vi "TDMS - File Viewer_Will.vi"(4 "error in (no error)":errorcluster, 7 "file path":path) -> (0 "error out":errorcluster, 3 "file path out":path)   [LabVIEW 2011]
doc: "Opens the .tdms file specified in the <B>file path</B> input and presents the file data in the TDMS File Viewer dialog box."
uses:
  <vilib>/Utility/tdmsutil.llb/fileViewerConfigData.ctl
  <vilib>/Utility/error.llb/DialogType.ctl
  <vilib>/Utility/tdmsutil.llb/TDMSFileViewerLocalizedText.vi
  Instance           1 26Saved   TDMS - File Viewer .vi
panel:
  in  "Help":bool
  in  "Status":string
  in  "Quit":bool
  in  "Settings...":bool
  in  "Properties / Values / Graph":T1(tab)
  in  "Properties":i32(listbox)
  in  "Raw data values":i32(listbox)
  out "Waveform Graph":waveform(dbl)[](graph)
  in  "File contents":string(tree)
  # "Displaying values 1..1000"
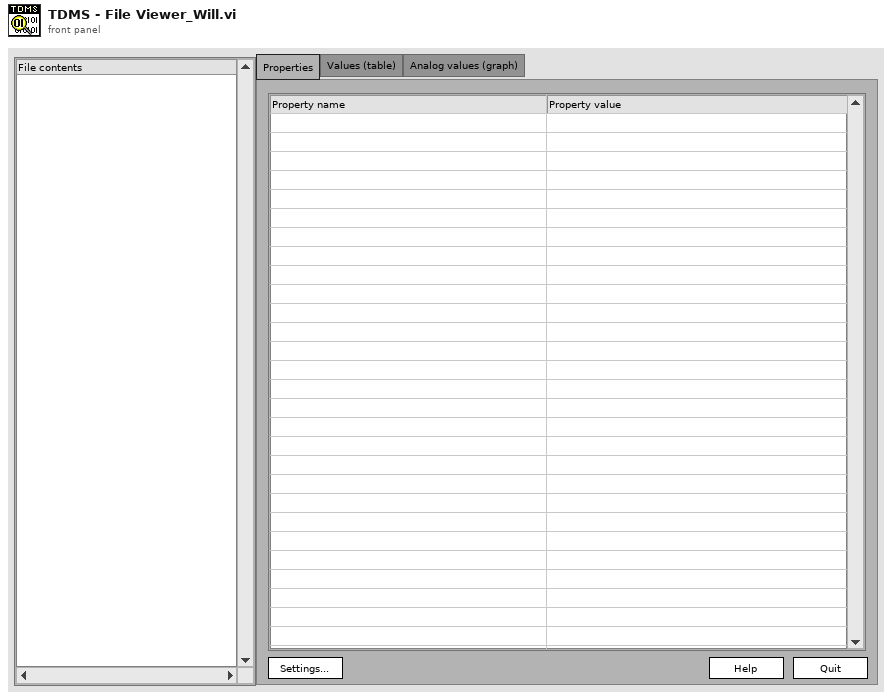
[diagram p1: front panel]
types:
  T1 = enum32{"Properties", "Values (table)", "Analog values (graph)"}
  T2 = enum16{"open", "open or create", "create or replace", "create", "open (read-only)"}
  T3 = cluster{"Tree":refnum<vi>, "Tab Control":refnum<vi>, "property list":refnum<vi>, "raw data list":refnum<vi>, "Waveform Graph":refnum<vi>, "Ok":refnum<vi>, "Ok 2":refnum<vi>, "Ok 3":refnum<vi>, "Ok 4":refnum<vi>}
  T4 = typedef "fileViewerConfigData.ctl" = cluster{"Show all (table)":bool, "Show all (graph)":bool, "limit (table)":u64, "limit (graph)":u64, "no show":bool, "start (table)":u64, "start (graph)":u64}
  T5 = typedef "DialogType.ctl" = u16
  T6 = typedef "LVRectTypeDef.ctl" = cluster{"left":i16, "top":i16, "right":i16, "bottom":i16}
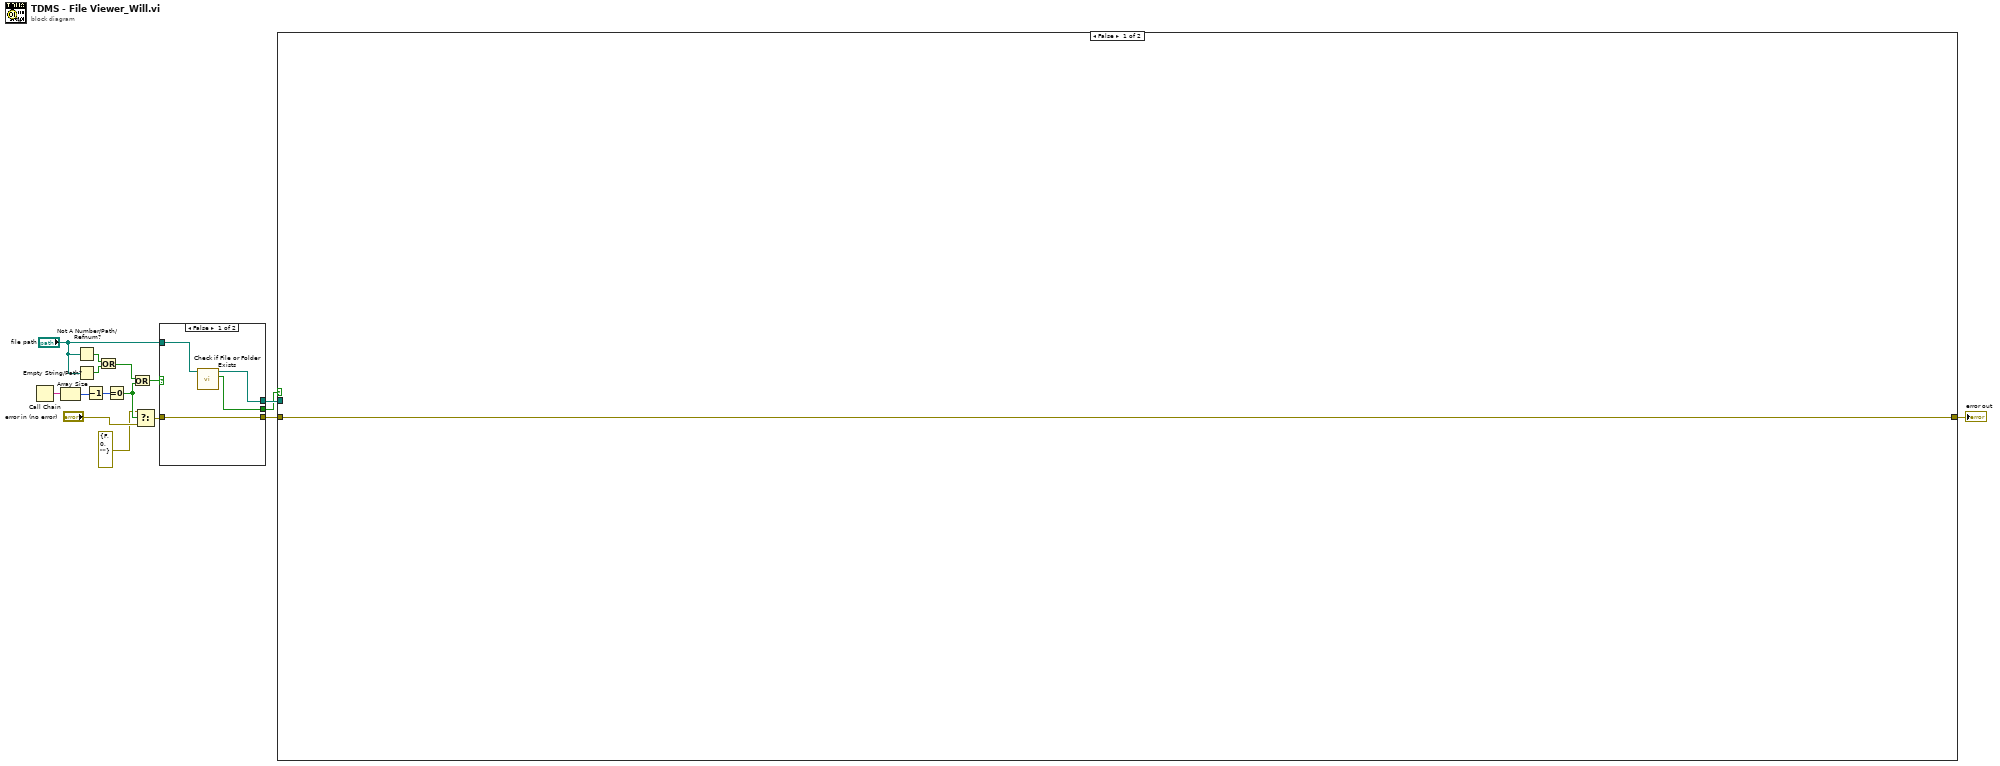
[diagram p0: block diagram]
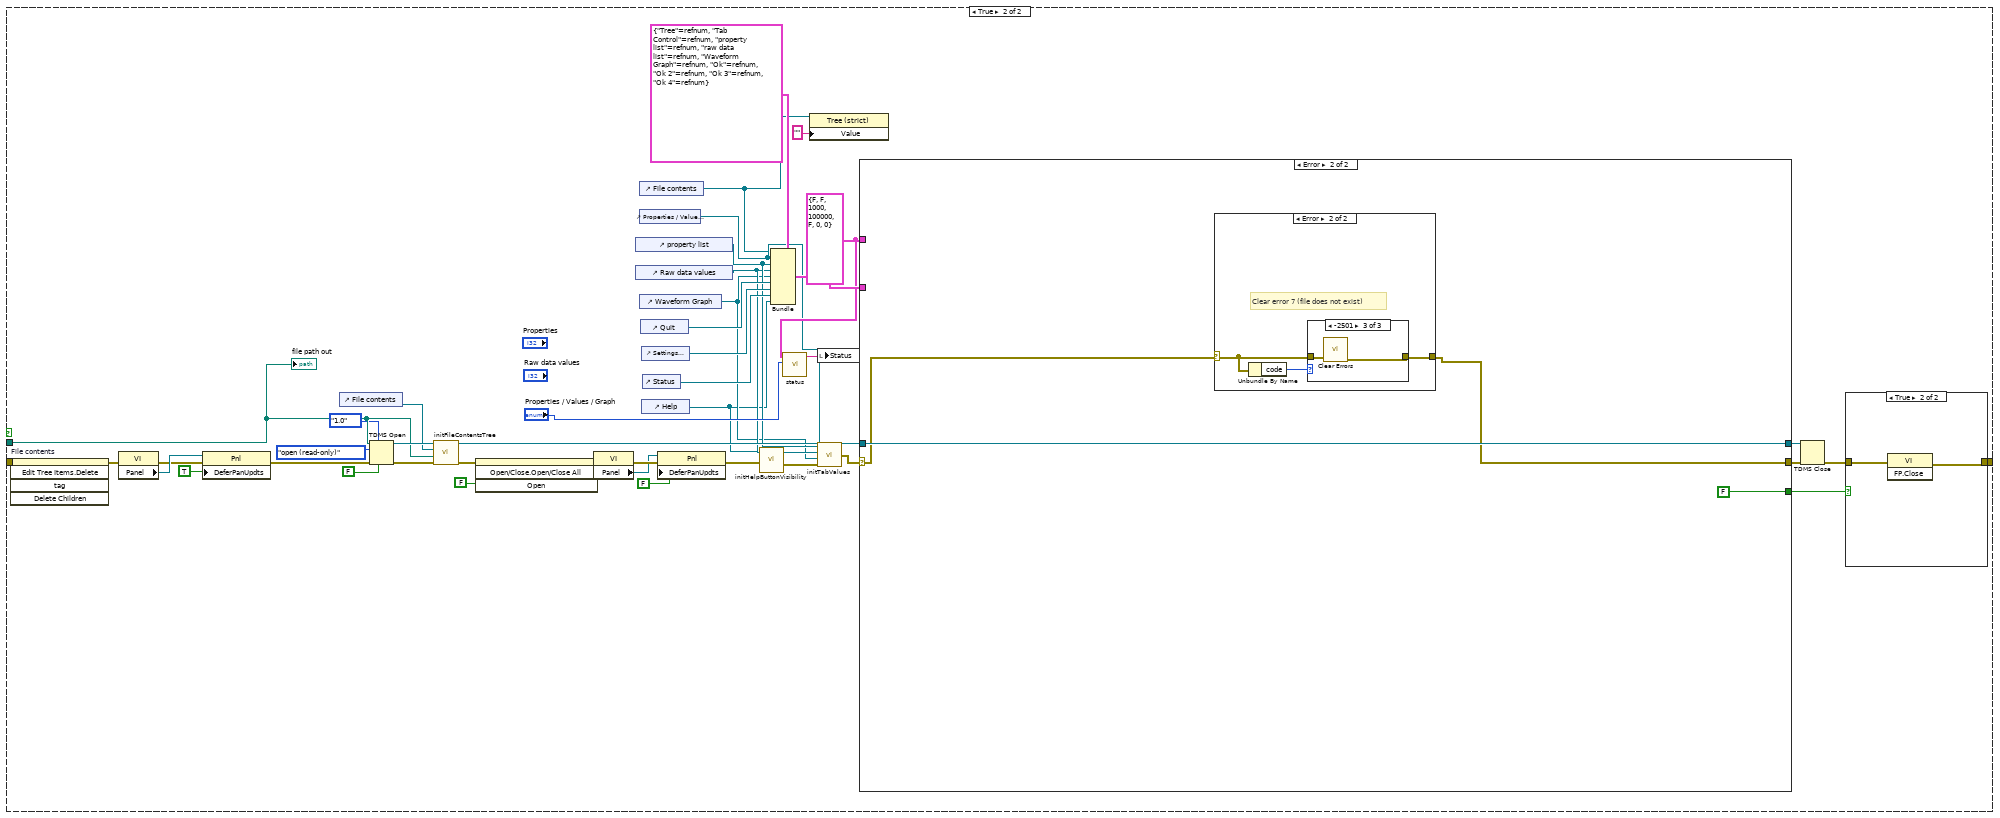
[diagram p2: hidden frame]
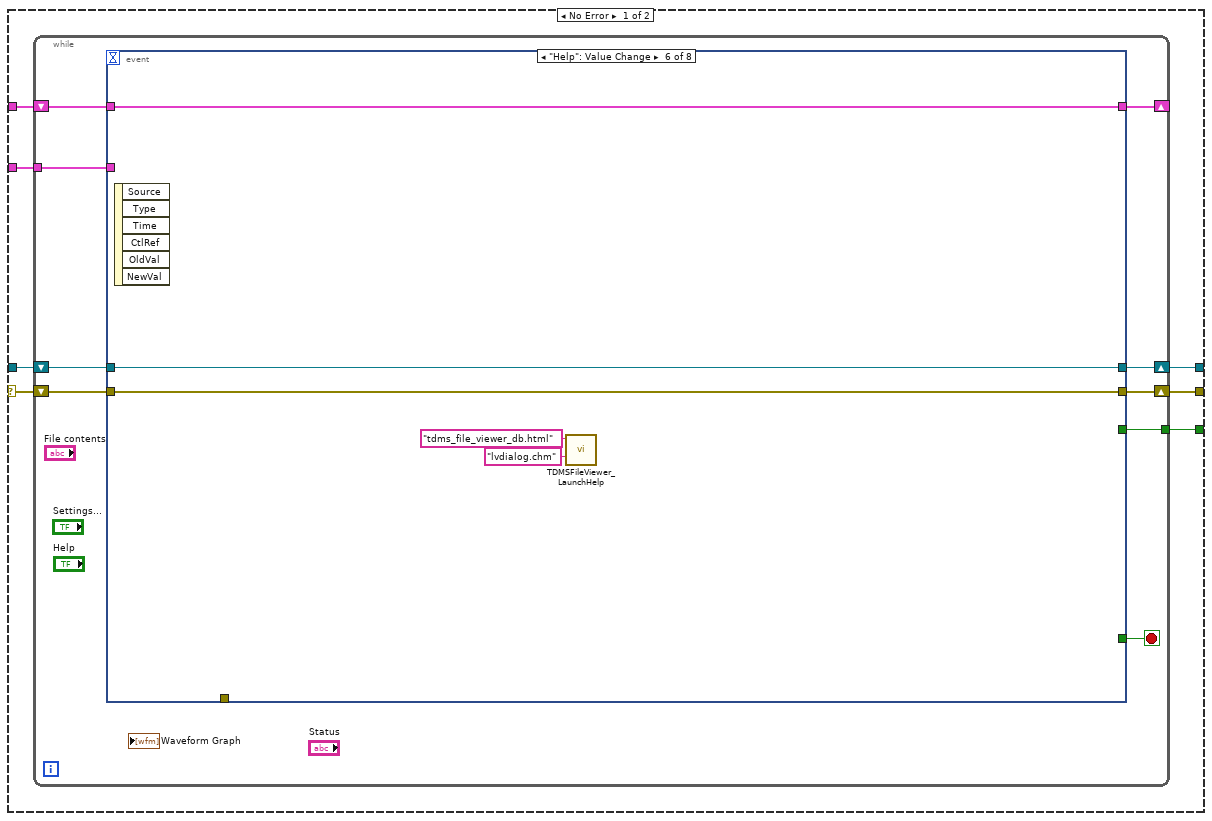
[diagram p4: hidden frame]
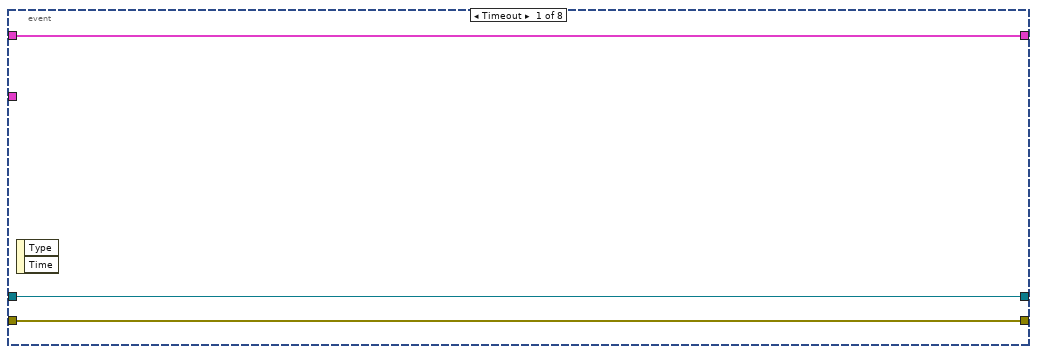
[diagram p5: hidden frame]
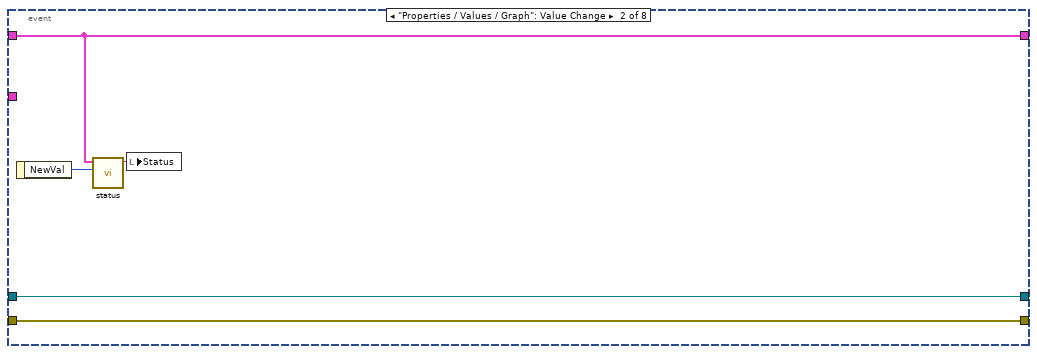
[diagram p6: hidden frame]
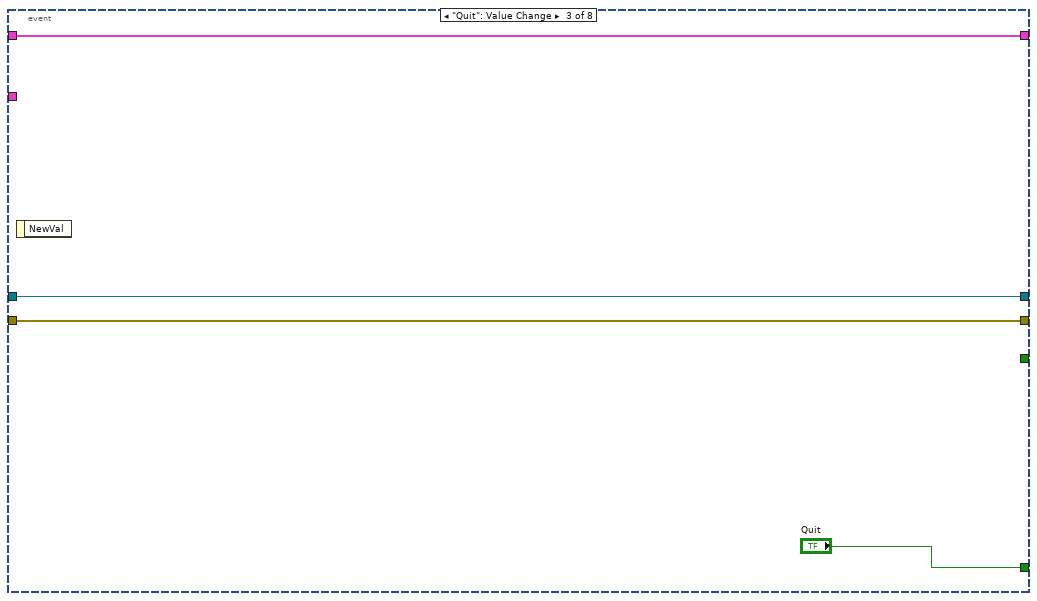
[diagram p7: hidden frame]
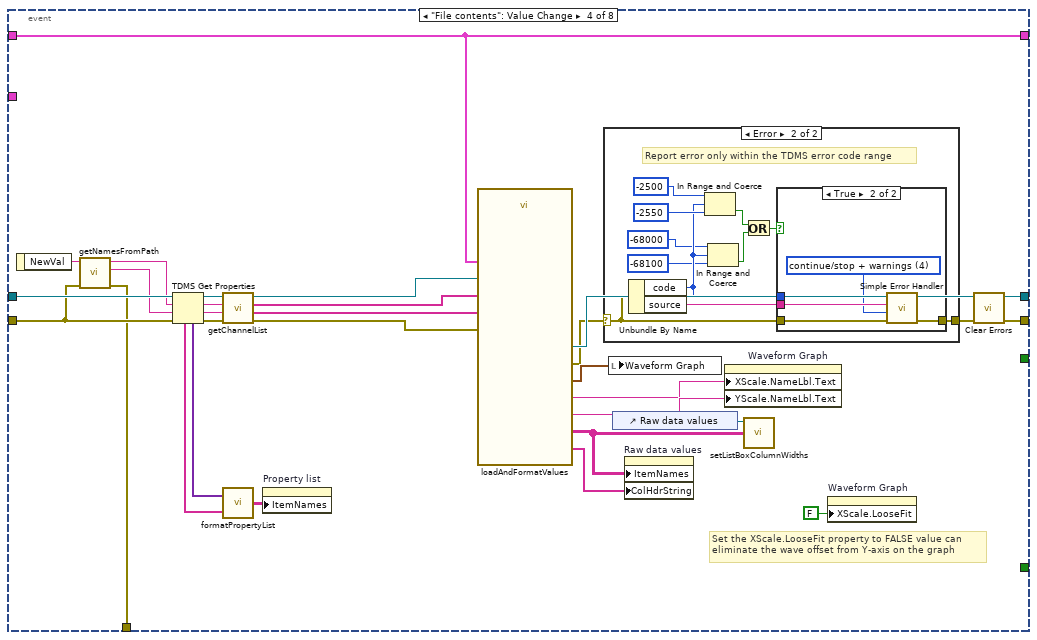
[diagram p8: hidden frame]
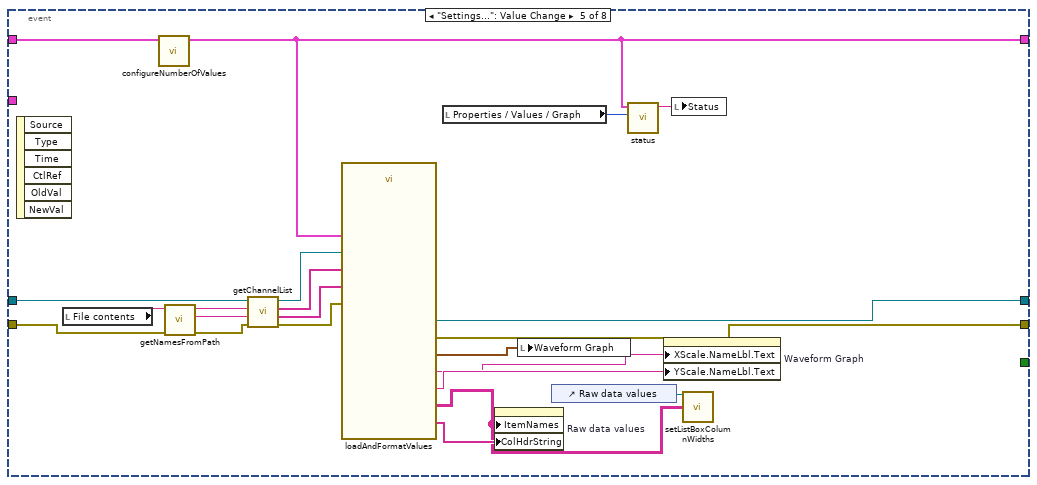
[diagram p11: hidden frame]
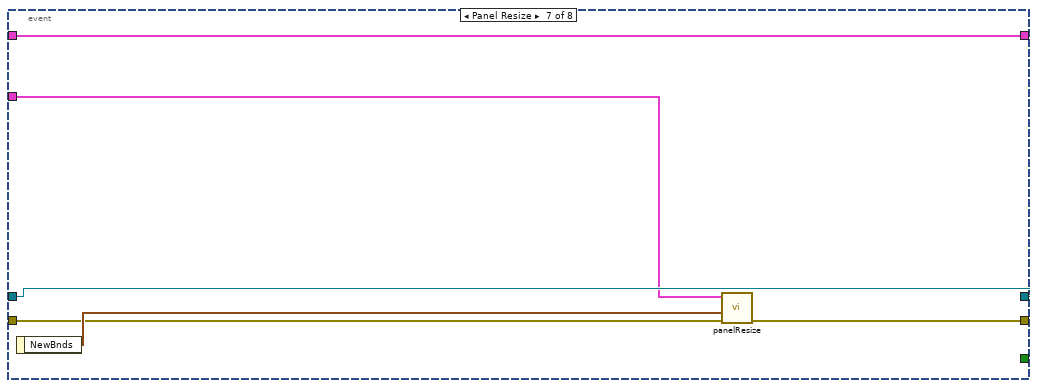
[diagram p12: hidden frame]
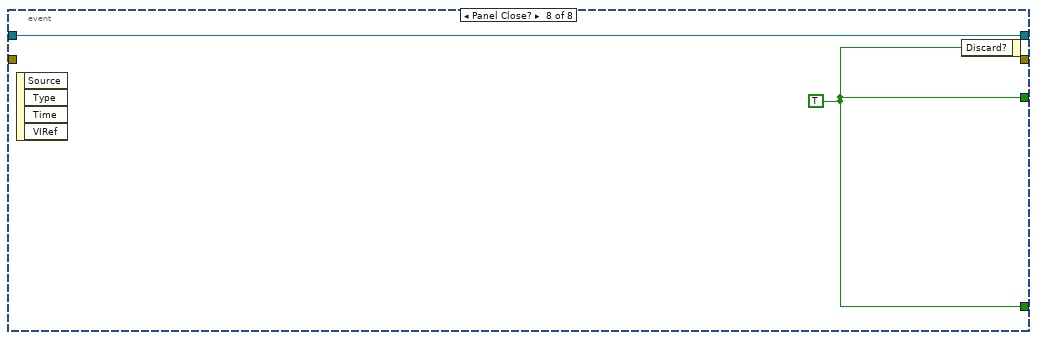
[diagram p13: hidden frame]
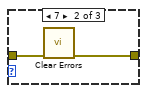
[diagram p16: hidden frame]
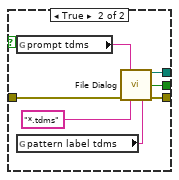
[diagram p17: hidden frame]
diagram:
  n1 = Call Chain() -> (call chain=w13:string[])
  n2 = Array Size(array=w13) -> (size(s)=w11:i32)
  n3 = Not A Number/Path/Refnum?(number/path/refnum="file path") -> (NaN/Path/Refnum?=w15:bool)
  n4 = Empty String/Path?(string/path="file path") -> (empty?=w14:bool)
  n5 = Decrement(x=w11) -> (x-1=w10:i32)
  n6 = Or(x=w15, y=w14) -> (x .or. y?=w12:bool)
  n7 = Equal To 0?(x=w10) -> (x = 0?=w6:bool)
  n8 = Or(x=w12, y=w6) -> (x .or. y?=w9:bool)
  n9 = Select(t=errorcluster {"status"=FALSE, "code"=0, "source"=""}, s=w6, f="error in (no error)") -> (s? t:f=w5:errorcluster)
  n10 = case shown="False" w9 {
    tunnel: [w18 w27] -> w8
    tunnel: "file path" -> [w19 _]
    tunnel: [w20 w25] -> w7
    tunnel: w5 -> [w20 w24]
    tunnel: [w17 w21] -> w1
    frame False {
      n11 = call <vilib>:"Check if File or Folder Exists.vi"("path"=w19) -> ("file or folder exists?"=w17:bool, "dup path"=w18:path)  [unwired: 8 in, 1 out]
    }
    frame True {
      n12 = global read "TDMSFileViewerLocalizedText.vi" "prompt tdms"() -> (w23:string)
      n13 = global read "TDMSFileViewerLocalizedText.vi" "pattern label tdms"() -> (w22:string)
      n14 = call "File Dialog"("prompt"=w23, "error in"=w24, "pattern (all files)"="*.tdms", "pattern label"=w22) -> ("selected path"=w27:path, "exists"=w21:bool, "error out"=w25:errorcluster)  [unwired: 3 in, 6 out]
    }
  }
  n15 = case shown="False" w1 {
    tunnel: w8 -> [_ w49]
    tunnel: w7 -> [w28 w48]
    tunnel: [w28 w41] -> w2
    frame False {
    }
    frame True {
      w45 = T4 {"Show all (table)"=FALSE, "Show all (graph)"=FALSE, "limit (table)"=1000, "limit (graph)"=100000, "no show"=FALSE, "start (table)"=0, "start (graph)"=0} ("TDMS File Viewer Configuration")
      n16 = invoke on="File contents" class="Tree (strict)" method="Edit Tree Items.Delete"(error in=w48) -> (error out=w62:errorcluster)  [unwired: 4 in, 4 out]
      n17 = property class="VI"(error in=w62) -> (error out=w63:errorcluster, "Panel"=w64:refnum<vi>)  [unwired: 1 in, 1 out]
      n18 = property class="Pnl"(reference=w64, error in=w63, "DeferPanUpdts"=TRUE ("Defer Panel Updates")) -> (error out=w66:errorcluster)  [unwired: 1 out]
      n19 = control-ref of="File contents"() -> (w50:refnum<vi>)
      n20 = TDMS Open(6:FALSE ("disable buffering (T)"), 7:enum16{"1.0", "2.0"}."1.0" ("file format version (2.0)"), 8:w66, 10:T2."open (read-only)" ("operation"), 11:w49) -> (0:w71:errorcluster, 3:w70:refnum<k34>)  [unwired: 1 in]
      n21 = call <vilib>:"initFileContentsTree.vi"("error in (no error)"=w71, "file path"=w49, "Tree Refnum"=w50, "tdms file"=w70) -> ("error out"=w58:errorcluster, "tdms file out"=w69:refnum<k34>)  [unwired: 2 out]
      n22 = invoke on="File contents" class="Tree (strict)" method="Open/Close.Open/Close All"(error in=w58, "Open"=FALSE ("Open?")) -> (error out=w57:errorcluster)  [unwired: 2 in, 3 out]
      n23 = property class="VI"(error in=w57) -> (error out=w60:errorcluster, "Panel"=w59:refnum<vi>)  [unwired: 1 in, 1 out]
      n24 = control-ref of="property list"() -> (w37:refnum<vi>)
      n25 = control-ref of="Raw data values"() -> (w36:refnum<vi>)
      n26 = control-ref of="Properties / Values / Graph"() -> (w34:refnum<vi>)
      n27 = control-ref of="Waveform Graph"() -> (w35:refnum<vi>)
      n28 = control-ref of="File contents"() -> (w33:refnum<vi>)
      n29 = control-ref of="Quit"() -> (w54:refnum<vi>)
      n30 = control-ref of="Settings..."() -> (w52:refnum<vi>)
      n31 = control-ref of="Help"() -> (w29:refnum<vi>)
      n32 = control-ref of="Status"() -> (w47:refnum<vi>)
      n33 = property class="Pnl"(reference=w59, error in=w60, "DeferPanUpdts"=FALSE ("Defer Panel Updates")) -> (error out=w31:errorcluster)  [unwired: 1 out]
      n34 = call <vilib>:"initHelpButtonVisibility.vi"("error in"=w31, "Help"=w29) -> ("error out"=w30:errorcluster)  [unwired: 9 in]
      n35 = Bundle(cluster=T3 {"Tree"=refnum, "Tab Control"=refnum, "property list"=refnum, "raw data list"=refnum, "Waveform Graph"=refnum, "Ok"=refnum, "Ok 2"=refnum, "Ok 3"=refnum, "Ok 4"=refnum} ("control refs"), "Tree"=w33, "Tab Control"=w34, "property list"=w37, "raw data list"=w36, "Waveform Graph"=w35, "Ok"=w54, "Ok 2"=w52, "Ok 3"=w47, "Ok 4"=w29) -> (w55:T3)
      n36 = call <vilib>:"status.vi"("tab sheet"="Properties / Values / Graph", "TDMS File Viewer Configuration"=w45) -> ("status"=w46:string)  [unwired: 5 out]
      n37 = property class="Tree (strict)"(reference=w33, "Value"="") -> ()  [unwired: 1 in, 2 out]
      n38 = local write "Status"(w46) -> ()
      n39 = call <vilib>:"initTabValues.vi"("properties"=w37, "Values"=w36, "waveform"=w35, "error in"=w30, "Properties / Values / Graph"=w34) -> ("error out"=w38:errorcluster)
      n40 = case shown="Error" w38 {
        selector: w38 -> [w76 w186]
        tunnel: w69 -> [w81 w188]
        tunnel: [w80 w188] -> w68
        tunnel: [w79 w185] -> w67
        tunnel: w55 -> [w78 _]
        tunnel: w45 -> [w77 _]
        tunnel: [w75 FALSE] -> w43
        frame No Error {
          n41 = while {
            shift-right: [w88] -> w79
            shift-left: w76 -> [w89]
            shift-right: [w87] -> w80
            shift-left: w81 -> [w90]
            tunnel: w78 -> [w85]
            shift-right: [w83] -> _
            shift-left: w77 -> [w84]
            tunnel: [w82] -> w75
            stop <- w86 stop-if-true
            n42 = event shown="[5] \"Help\": Value Change" {
              selector: _ -> [_ _ _ _ _ _ _ _]
              dyn-events: _ -> [_ _ _ _ _ _ _ _]
              timeout: _ -> [_ _ _ _ _ _ _ _]
              tunnel: w90 -> [w92 w97 w101 w131 w160 w175 w182 w184]
              tunnel: w89 -> [w93 w98 w100 w123 w168 w174 w179 _]
              tunnel: [w93 w98 w100 w119 w169 w174 w178 _] -> w88
              tunnel: [w92 w97 w101 w130 w170 w175 w182 w184] -> w87
              tunnel: [_ _ "Quit" _ _ _ _ w183] -> w86
              tunnel: [_ _ _ w122 _ _ _ _] -> _
              tunnel: w85 -> [_ _ _ _ _ _ w180 _]
              tunnel: w84 -> [w91 w94 w99 w112 w171 w176 w177 _]
              tunnel: [w91 w94 w99 w112 w150 w176 w177 _] -> w83
              tunnel: [_ _ _ _ _ _ _ w183] -> w82
              event Timeout {
                n43 = event-data() -> ()  [unwired: 3 out]
              }
              event "Properties / Values / Graph": Value Change {
                n44 = event-data() -> ("NewVal"=w96:T1)  [unwired: 1 out]
                n45 = call <vilib>:"status.vi"("tab sheet"=w96, "TDMS File Viewer Configuration"=w94) -> ("status"=w95:string)  [unwired: 5 out]
                n46 = local write "Status"(w95) -> ()
              }
              event "Quit": Value Change {
                n47 = event-data() -> ()  [unwired: 2 out]
              }
              event "File contents": Value Change {
                # "Set the XScale.LooseFit property to FALSE value can \neliminate the wave offset from Y-axis on the graph"
                n48 = event-data() -> ("NewVal"=w125:string)  [unwired: 1 out]
                n49 = call <vilib>:"getNamesFromPath.vi"("error in (no error)"=w123, "tree path"=w125) -> ("error out"=w122:errorcluster, "channel"=w128:string, "group"=w129:string)  [unwired: 3 out]
                n50 = TDMS Get Properties(8:w123, 9:w128, 10:w129, 11:w131) -> (0:w117:errorcluster, 1:w116:string, 2:w110:string, 3:w118:refnum<k34>, 4:w126:variant[], 6:w127:string[])  [unwired: 2 out]
                n51 = call <vilib>:"getChannelList.vi"("error in (no error)"=w117, "channel names"=w116, "group name"=w110, "tdms file"=w118) -> ("error out"=w106:errorcluster, "channel names out"=w107:string[], "group names out"=w108:string[], "tdms file out"=w109:refnum<k34>)
                n52 = call <vilib>:"formatPropertyList.vi"("property names"=w127, "property values"=w126) -> ("strings"=w124:string[][])
                n53 = property on="Property list" class="MCListbox (strict)"("ItemNames"=w124) -> ()  [unwired: 2 in, 2 out]
                n54 = call <vilib>:"loadAndFormatValues.vi"("error in (no error)"=w106, "configuration"=w112, "channel names"=w107, "group names"=w108, "tdms file"=w109) -> ("error out"=w105:errorcluster, "graph y names"=w114:string, "graph x names"=w113:string, "tdms file out"=w130:refnum<k34>, "waveform values"=w111:waveform(dbl)[], "table values"=w121:string[][], "table headers"=w115:string[])
                n55 = case shown="Error" w105 {
                  selector: w105 -> [w132 w142]
                  tunnel: [w132 w141] -> w104
                  frame No Error {
                  }
                  frame Error {
                    # "Report error only within the TDMS error code range"
                    n56 = Unbundle By Name(w142) -> ("code"=w138:i32, "source"=w143:string)
                    n57 = In Range and Coerce(upper limit=-2500, x=w138, lower limit=-2550 ("upper limit")) -> (In Range?=w135:bool)  [unwired: 1 out]
                    n58 = In Range and Coerce(upper limit=-68000, x=w138, lower limit=-68100) -> (In Range?=w134:bool)  [unwired: 1 out]
                    n59 = Or(x=w135, y=w134) -> (x .or. y?=w133:bool)
                    n60 = case shown="True" w133 {
                      tunnel: w143 -> [_ w149]
                      tunnel: w142 -> [w144 w148]
                      tunnel: [w144 w147] -> w141
                      tunnel: w138 -> [_ w145]
                      frame False {
                        # "Out of the range of TDMS\nerror code, we don't report\nthem."
                      }
                      frame True {
                        w146 = T5 4 items=["no dialog", "OK message", "continue or stop message", "OK message + warnings", "continue/stop + warnings"] ("type of dialog (OK msg:1)")
                        n61 = call <vilib>:"Simple Error Handler.vi"("error code (no error:0)"=w145, "error source (\" \")"=w149, "type of dialog (OK msg:1)"=w146, "error in (no error)"=w148) -> ("error out"=w147:errorcluster)  [unwired: 1 in, 4 out]
                      }
                    }
                  }
                }
                n62 = local write "Waveform Graph"(w111) -> ()
                n63 = control-ref of="Raw data values"() -> (w120:refnum<vi>)
                n64 = property on="Raw data values" class="MCListbox (strict)"("ItemNames"=w121, "ColHdrString"=w115) -> ()  [unwired: 2 in, 2 out]
                n65 = property on="Waveform Graph" class="WFGraph (strict)"("XScale.NameLbl.Text"=w113, "YScale.NameLbl.Text"=w114) -> ()  [unwired: 2 in, 2 out]
                n66 = call <vilib>:"setListBoxColumnWidths.vi"("table data"=w121, "MCListbox Refnum"=w120) -> ()  [unwired: 1 out]
                n67 = property on="Waveform Graph" class="WFGraph (strict)"("XScale.LooseFit"=FALSE ("X Scale.Loose Fit")) -> ()  [unwired: 2 in, 2 out]
                n68 = call <vilib>:"Clear Errors.vi"("error in (no error)"=w104) -> ("error out"=w119:errorcluster)  [unwired: 6 out]
              }
              event "Settings...": Value Change {
                n69 = event-data() -> ()  [unwired: 7 out]
                n70 = local read "File contents"() -> (w161:string)
                n71 = call <vilib>:"configureNumberOfValues.vi"("TDMS File Viewer Configuration"=w171) -> ("TDMS File Viewer Configuration Out"=w150:T4)  [unwired: 10 out]
                n72 = call <vilib>:"getNamesFromPath.vi"("error in (no error)"=w168, "tree path"=w161) -> ("error out"=w159:errorcluster, "channel"=w157:string, "group"=w158:string)  [unwired: 3 out]
                n73 = call <vilib>:"getChannelList.vi"("error in (no error)"=w159, "channel names"=w157, "group name"=w158, "tdms file"=w160) -> ("error out"=w156:errorcluster, "channel names out"=w153:string[], "group names out"=w154:string[], "tdms file out"=w155:refnum<k34>)
                n74 = call <vilib>:"loadAndFormatValues.vi"("error in (no error)"=w156, "configuration"=w150, "channel names"=w153, "group names"=w154, "tdms file"=w155) -> ("error out"=w169:errorcluster, "graph y names"=w163:string, "graph x names"=w162:string, "tdms file out"=w170:refnum<k34>, "waveform values"=w167:waveform(dbl)[], "table values"=w164:string[][], "table headers"=w166:string[])
                n75 = local read "Properties / Values / Graph"() -> (w151:T1)
                n76 = property on="Raw data values" class="MCListbox (strict)"("ItemNames"=w164, "ColHdrString"=w166) -> ()  [unwired: 2 in, 2 out]
                n77 = local write "Waveform Graph"(w167) -> ()
                n78 = control-ref of="Raw data values"() -> (w165:refnum<vi>)
                n79 = call <vilib>:"status.vi"("tab sheet"=w151, "TDMS File Viewer Configuration"=w150) -> ("status"=w152:string)  [unwired: 5 out]
                n80 = property on="Waveform Graph" class="WFGraph (strict)"("XScale.NameLbl.Text"=w162, "YScale.NameLbl.Text"=w163) -> ()  [unwired: 2 in, 2 out]
                n81 = local write "Status"(w152) -> ()
                n82 = call <vilib>:"setListBoxColumnWidths.vi"("table data"=w164, "MCListbox Refnum"=w165) -> ()  [unwired: 1 out]
              }
              event "Help": Value Change {
                n83 = event-data() -> ()  [unwired: 7 out]
                n84 = call <vilib>:"TDMSFileViewer_LaunchHelp.vi"("CHM or HLP filename (lvdialog.chm)"="lvdialog.chm", "HTML filename"="tdms_file_viewer_db.html") -> ()  [unwired: 1 in, 5 out]
              }
              event Panel Resize {
                n85 = event-data() -> ("NewBnds"=w181:T6)  [unwired: 1 out]
                n86 = call <vilib>:"panelResize.vi"("error in (no error)"=w179, "NewBnds"=w181, "control refs"=w180) -> ("error out"=w178:errorcluster)  [unwired: 4 in]
              }
              event Panel Close? {
                w183 = TRUE
                n87 = event-data() -> ()  [unwired: 5 out]
                n88 = event-data("Discard?"=w183) -> ()  [unwired: 1 in, 1 out]
              }
            }
          }
        }
        frame Error {
          n89 = case shown="Error" w186 {
            selector: w186 -> [w189 w191]
            tunnel: [w189 w190] -> w185
            frame No Error {
            }
            frame Error {
              # "Clear error 7 (file does not exist)"
              n90 = Unbundle By Name(w191) -> ("code"=w192:i32)
              n91 = case shown="-2501" w192 {
                tunnel: w191 -> [w193 w195 w197]
                tunnel: [w193 w194 w196] -> w190
                frame Default {
                }
                frame 7 {
                  n92 = call <vilib>:"Clear Errors.vi"("error in (no error)"=w195) -> ("error out"=w194:errorcluster)  [unwired: 6 in]
                }
                frame -2501 {
                  n93 = call <vilib>:"Clear Errors.vi"("error in (no error)"=w197) -> ("error out"=w196:errorcluster)  [unwired: 6 in]
                }
              }
            }
          }
        }
      }
      n94 = TDMS Close(8:w67, 11:w68) -> (0:w42:errorcluster)  [unwired: 1 out]
      n95 = case shown="True" w43 {
        tunnel: w42 -> [w72 w74]
        tunnel: [w72 w73] -> w41
        frame False {
        }
        frame True {
          n96 = invoke class="VI" method="FP.Close"(error in=w74) -> (error out=w73:errorcluster)  [unwired: 2 in, 2 out]
        }
      }
      "file path out" <- w49
    }
  }
  "error out" <- w2
